vi "projekt.vi"() -> ()   [LabVIEW 2022 SP3]
uses:
  <vilib>/Instr/_visa.llb/VISA Configure Serial Port (Instr).vi
  <vilib>/Utility/file.llb/Write Delimited Spreadsheet (string).vi
  <vilib>/Utility/file.llb/Write Delimited Spreadsheet (DBL).vi
  <vilib>/addons/control/pid/pid.llb/PID (DBL).vi
  <vilib>/addons/control/pid/NI_PID_pid.lvlib
panel:
  in  "file path (dialog if empty)":path=path "D:/IS/Sławomir Klimowski & Karolina Kotlowska/projekt/temperature.txt"
  out "Square function fill":cluster{dbl[], dbl[]}(graph)
  out "Heating element state":cluster{dbl[], dbl[]}(graph)
  out "Temperature":cluster{dbl[], dbl[]}[](graph)
  in  "Temperature":dbl=22.0 format="%.2f"
  out "output 1":dbl
  in  "Stop program":bool
  out "read buffer (debug)":string
  in  "VISA resource name":refnum<visa-resource-name>
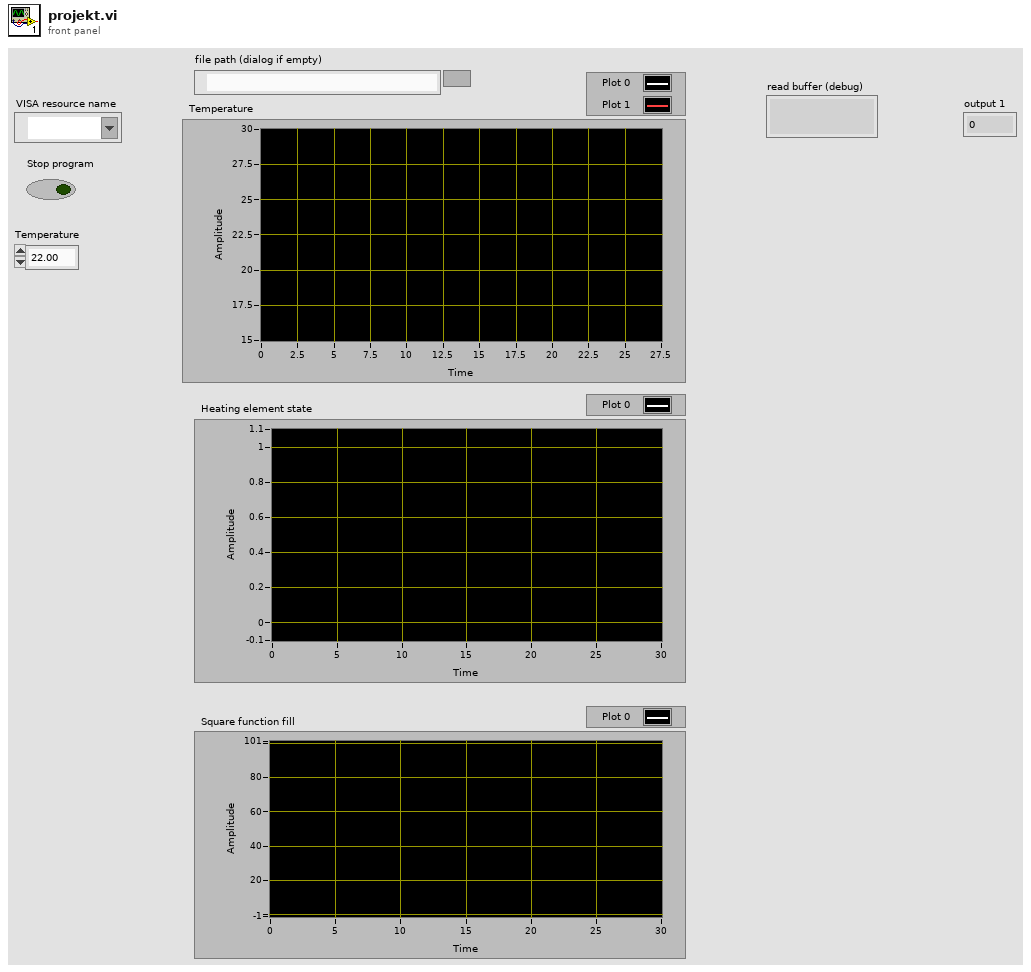
[diagram p1: front panel]
types:
  T1 = cluster{"proportional gain (Kc)":dbl, "integral time (Ti, min)":dbl, "derivative time (Td, min)":dbl}
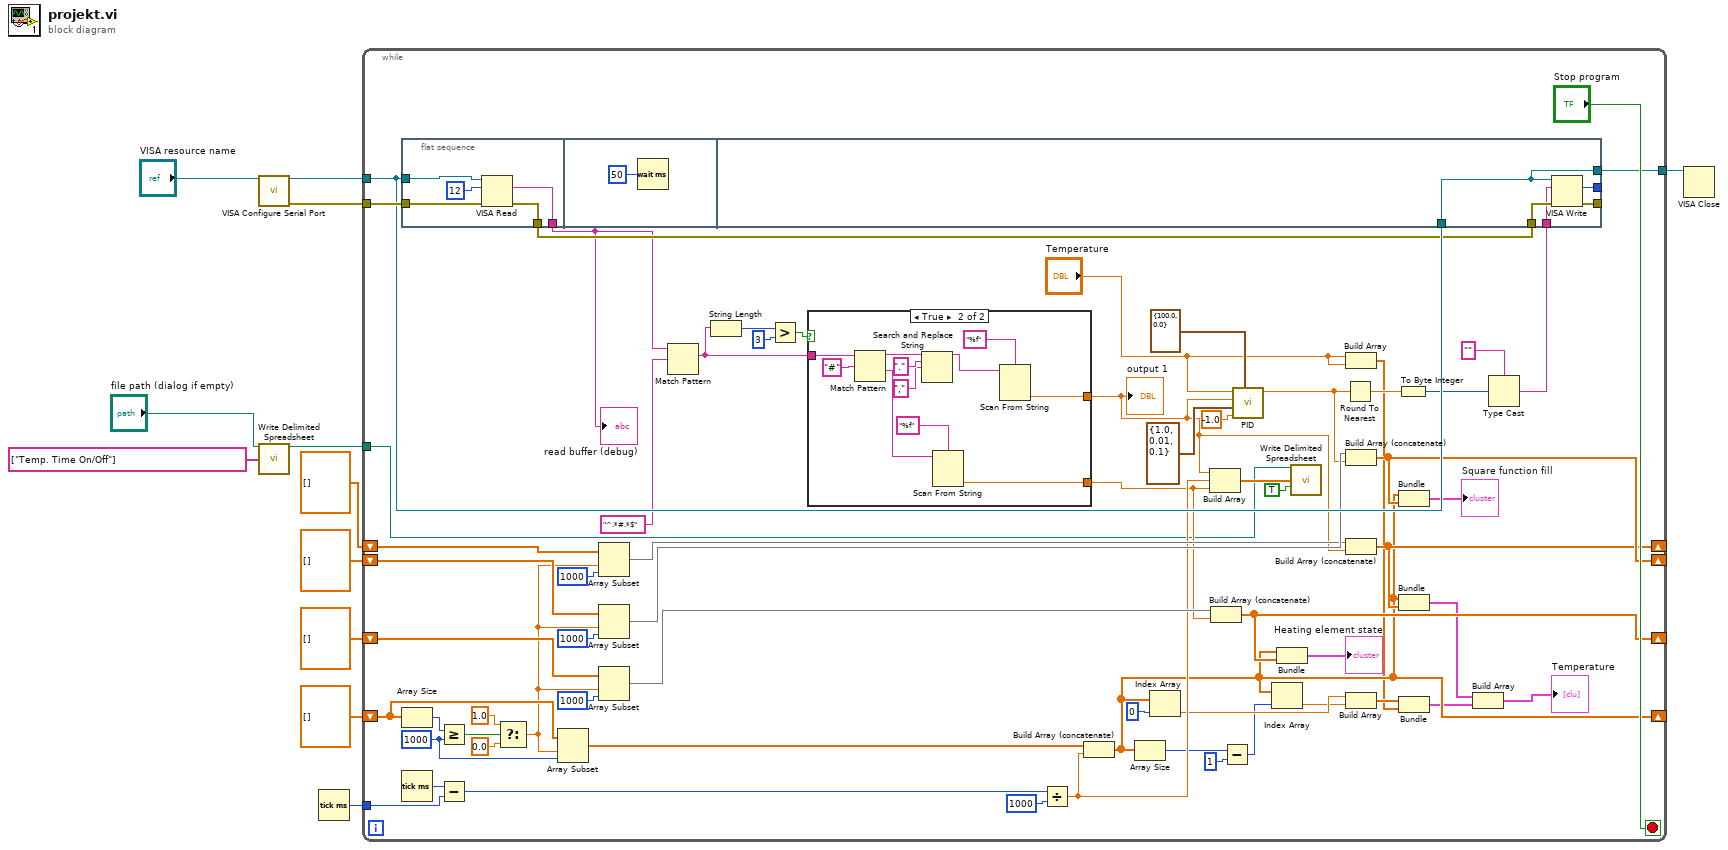
[diagram p0: block diagram]
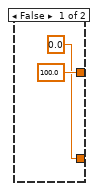
[diagram p2: hidden frame]
diagram:
  n1 = call-poly "VISA Configure Serial Port"("VISA resource name"="VISA resource name") -> ("VISA resource name out"=w11:refnum<visa-resource-name>, "error out"=w10:errorcluster)  [unwired: 13 in]
  n2 = call-poly <vilib>:"Write Delimited Spreadsheet.vi"("file path (dialog if empty)"="file path (dialog if empty)", "1D data"=string[] ["Temp. Time On/Off"]) -> ("new file path (Not A Path if cancelled)"=w2:path)  [unwired: 12 in, 1 out]
  n3 = Tick Count (ms)() -> (millisecond timer value=w9:u32)
  n4 = while {
    tunnel: w11 -> [w71]
    tunnel: w10 -> [w72]
    tunnel: w9 -> [w62]
    shift-right: [w18] -> _
    shift-left: dbl[] [] -> [w42]
    shift-right: [w47] -> _
    shift-left: dbl[] [] -> [w45]
    shift-right: [w48] -> _
    shift-left: dbl[] [] -> [w50]
    shift-right: [w53] -> _
    shift-left: dbl[] [] -> [w54]
    tunnel: [w35] -> w4
    tunnel: w2 -> [w26]
    stop <- "Stop program" stop-if-true
    w40 = 1000 ("length")
    n5 = flat-sequence {
      tunnel: w72 -> [w94]
      tunnel: w71 -> [w93]
      tunnel: [w92] -> w70
      tunnel: [w91] -> w69
      tunnel: w70 -> [w100]
      tunnel: w57 -> [w99]
      tunnel: w71 -> [w96]
      tunnel: [w97] -> _
      tunnel: [w98] -> _
      tunnel: [w96] -> w35
      frame #0 {
        n6 = VISA Read(VISA resource name=w93, byte count=u32 12, error in (no error)=w94) -> (read buffer=w91:string, error out=w92:errorcluster)  [unwired: 2 out]
      }
      frame #1 {
        n7 = Wait (ms)(milliseconds to wait=u32 50) -> ()  [unwired: 1 out]
      }
      frame #2 {
        n8 = VISA Write(VISA resource name=w96, write buffer=w99, error in (no error)=w100) -> (return count=w98:u32, error out=w97:errorcluster)  [unwired: 1 out]
      }
    }
    n9 = Array Size(array=w42) -> (size(s)=w41:i32)
    n10 = Tick Count (ms)() -> (millisecond timer value=w63:u32)
    n11 = Greater Or Equal?(x=w41, y=w40) -> (x >= y?=w39:bool)
    n12 = Subtract(x=w63, y=w62) -> (x-y=w61:u32)
    n13 = Select(t=1.0, s=w39, f=0.0) -> (s? t:f=w36:dbl)
    n14 = Array Subset(array=w42, index=w36, length=w40) -> (w43:dbl[])
    n15 = Array Subset(array=w45, index=w36, length=1000) -> (w44:dbl[])
    n16 = Array Subset(array=w54, index=w36, length=1000) -> (w52:dbl[])
    n17 = Array Subset(array=w50, index=w36, length=1000) -> (w49:dbl[])
    n18 = Match Pattern(string=w69, regular expression="^.*#.*$") -> (match substring=w64:string)  [unwired: 1 in, 3 out]
    n19 = String Length(string=w64) -> (length=w66:i32)
    n20 = Greater?(x=w66, y=3) -> (0:w65:bool)
    n21 = case shown="True" w65 {
      tunnel: [100.0 w84] -> w32
      tunnel: [0.0 w87] -> w27
      tunnel: w64 -> [_ w83]
      frame False {
      }
      frame True {
        n22 = Match Pattern(string=w83, regular expression="#") -> (before substring=w82:string, after substring=w86:string)  [unwired: 1 in, 2 out]
        n23 = Search and Replace String(input string=w82, search string=".", replace string="," ("replace string (\"\")")) -> (result string=w79:string)  [unwired: 5 in, 3 out]
        n24 = Scan From String(format string="%f", input string=w86) -> (output 1=w87:dbl)  [unwired: 3 in, 3 out]
        n25 = Scan From String(format string="%f", input string=w79) -> (output 1=w84:dbl)  [unwired: 3 in, 3 out]
      }
    }
    "output 1" <- w32
    n26 = Divide(x=w61, y=u32 1000) -> (x/y=w28:dbl)
    n27 = Build Array (concatenate)(w43, w28) -> (w18:dbl[])
    n28 = Array Size(array=w18) -> (size(s)=w22:i32)
    n29 = Index Array(array=w18, index=0) -> (element=w23:dbl)
    n30 = Build Array(w32, w28, w27) -> (w33:dbl[])
    n31 = Build Array (concatenate)(w49, w27) -> (w48:dbl[])
    n32 = Subtract(x=w22, y=1) -> (x-y=w20:i32)
    n33 = call-poly <vilib>:"PID.vi"("output range"=cluster{"output high":dbl, "output low":dbl} {"output high"=100.0, "output low"=0.0}, "dt (s)"=-1.0, "PID gains"=T1 {"proportional gain (Kc)"=1.0, "integral time (Ti, min)"=0.01, "derivative time (Td, min)"=0.1}, "process variable"=w32, "setpoint"="Temperature") -> ("output"=w34:dbl)  [unwired: 5 in, 1 out]
    n34 = Index Array(array=w18, index=w20) -> (element=w19:dbl)
    n35 = Bundle(w18, w48) -> (→"Heating element state":cluster{dbl[], dbl[]})  [unwired: 1 in]
    n36 = call-poly <vilib>:"Write Delimited Spreadsheet.vi"("file path (dialog if empty)"=w26, "1D data"=w33, "append to file? (new file:F)"=TRUE) -> ()  [unwired: 11 in, 2 out]
    n37 = Round To Nearest(number=w34) -> (nearest integer value=w29:dbl)
    n38 = Build Array("Temperature", "Temperature") -> (w16:dbl[])
    n39 = Build Array (concatenate)(w52, w34) -> (w53:dbl[])
    n40 = Build Array (concatenate)(w44, w32) -> (w47:dbl[])
    n41 = Build Array(w23, w19) -> (w17:dbl[])
    n42 = To Byte Integer(number=w29) -> (8bit integer=w30:i8)
    n43 = Bundle(w18, w53) -> (→"Square function fill":cluster{dbl[], dbl[]})  [unwired: 1 in]
    n44 = Bundle(w18, w47) -> (w15:cluster{dbl[], dbl[]})  [unwired: 1 in]
    n45 = Bundle(w17, w16) -> (w14:cluster{dbl[], dbl[]})  [unwired: 1 in]
    n46 = Build Array(w15, w14) -> (→"Temperature":cluster{dbl[], dbl[]}[])
    n47 = Type Cast(type="", x=w30) -> (*(type *) &x=w57:string)
    "read buffer (debug)" <- w69
  }
  n48 = VISA Close(VISA resource name=w4) -> ()  [unwired: 1 in, 1 out]
